vi "write correction factor.vi"() -> ()   [LabVIEW 2016]
uses:
  <vilib>/Utility/file.llb/Write Delimited Spreadsheet (DBL).vi
panel:
  in  "Other Factor":dbl[](array[numeric])
  in  "Cable Loss":dbl[](array[numeric])
  in  "Antenna Factor":dbl[](array[numeric])
  out "Appended Array":dbl[][](array[numeric])
  out "Concatenated Array":dbl[](array[numeric])
  in  "Other Frequency":dbl[](array[numeric])
  in  "Cable Frequency":dbl[](array[numeric])
  in  "Antenna Frequency":dbl[](array[numeric])
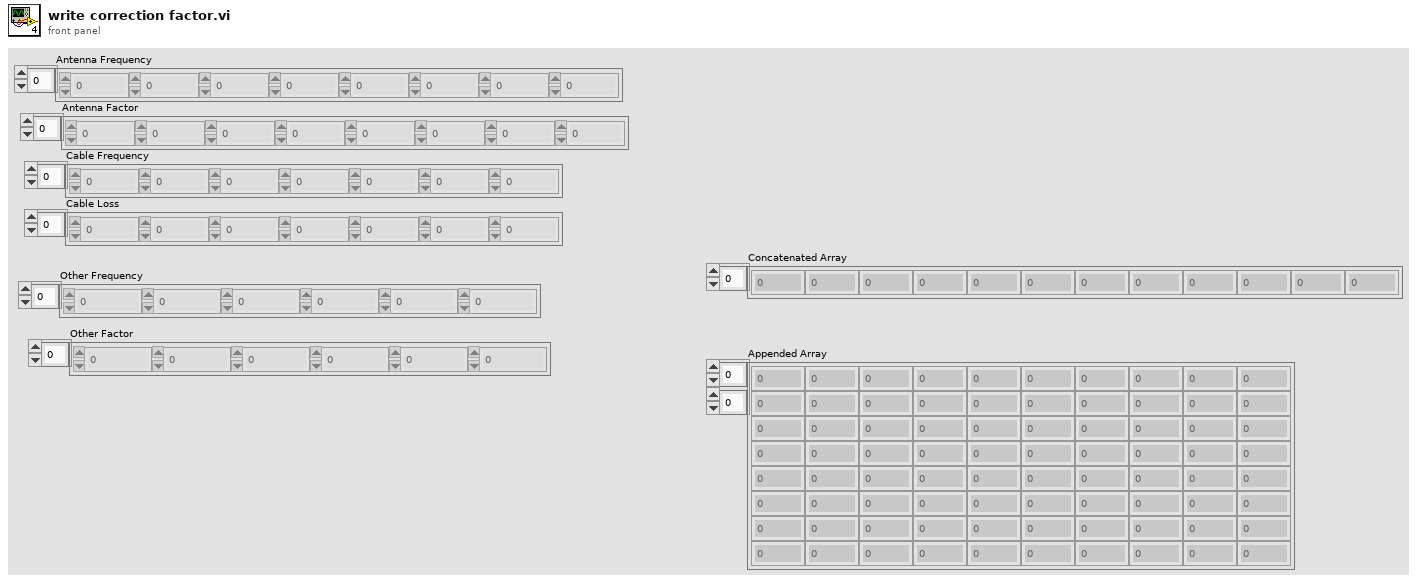
[diagram p1: front panel]
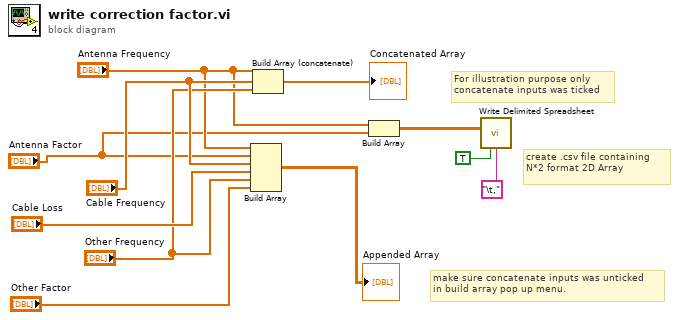
[diagram p0: block diagram]
diagram:
  # "create .csv file containing \nN*2 format 2D Array"
  # "make sure concatenate inputs was unticked\nin build array pop up menu."
  # "For illustration purpose only\nconcatenate inputs was ticked"
  n1 = Build Array("Antenna Frequency", "Antenna Factor", "Cable Frequency", "Cable Loss", "Other Frequency", "Other Factor") -> (→"Appended Array":dbl[][])
  n2 = Build Array (concatenate)("Antenna Frequency", "Cable Frequency", "Other Frequency") -> (→"Concatenated Array":dbl[])
  n3 = Build Array("Antenna Frequency", "Antenna Factor") -> (w1:dbl[][])
  n4 = call-poly <vilib>:"Write Delimited Spreadsheet.vi"("2D data"=w1, "transpose? (no:F)"=TRUE, "delimiter (\\t)"="\t," ("delimiter (\\t)")) -> ()  [unwired: 11 in, 2 out]
